vi "Untitled 2 (SubVI).vi"(7 "Disabled":T1(ring), 8 "error in (no error)":errorcluster, 11 "Array":refnum<vi>[](array[refnum])) -> (0 "error out":errorcluster)   [LabVIEW 2013]
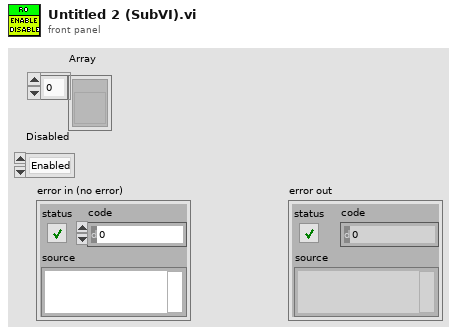
[diagram p1: front panel]
types:
  T1 = enum8{"Enabled", "Disabled", "Disabled and Grayed Out"}
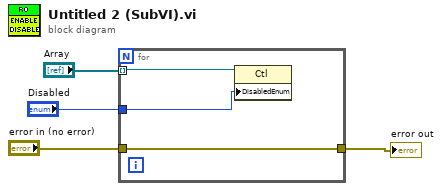
[diagram p0: block diagram]
diagram:
  n1 = for {
    tunnel: "Array" -> [w7] mode=indexing
    tunnel: [w6] -> w3
    tunnel: "error in (no error)" -> [w6]
    tunnel: "Disabled" -> [w5]
    n2 = property class="Ctl"(reference=w7, "DisabledEnum"=w5) -> ()  [unwired: 1 in, 2 out]
  }
  "error out" <- w3
